vi "Police panel.vi"() -> ()   [LabVIEW 2018]
panel:
  in  "Police Arrived 2":bool
  out "Accident":bool
  in  "Done":bool
  in  "Police Arrived":bool
  in  "Logout":bool
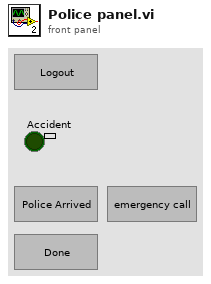
[diagram p1: front panel]
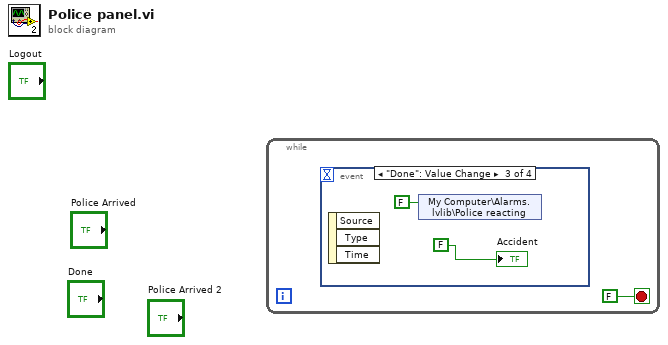
[diagram p0: block diagram]
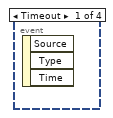
[diagram p2: hidden frame]
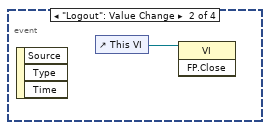
[diagram p3: hidden frame]
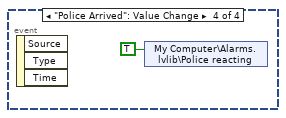
[diagram p4: hidden frame]
diagram:
  n1 = while {
    stop <- FALSE stop-if-true
    n2 = event shown="[2] \"Done\": Value Change" {
      selector: _ -> [_ _ _ _]
      dyn-events: _ -> [_ _ _ _]
      timeout: _ -> [_ _ _ _]
      event Timeout {
        n3 = event-data() -> ()  [unwired: 1 in, 3 out]
      }
      event "Logout": Value Change {
        n4 = event-data() -> ()  [unwired: 1 in, 3 out]
        n5 = control-ref of="This VI"() -> (w2:refnum<vi>)
        n6 = invoke class="VI" method="FP.Close"(reference=w2) -> ()  [unwired: 2 in, 3 out]
      }
      event "Done": Value Change {
        n7 = event-data() -> ()  [unwired: 1 in, 3 out]
        n8 = shared-variable "My Computer\\Alarms.lvlib\\Police reacting"(FALSE ("Repairing")) -> ()  [unwired: 1 in, 1 out]
        "Accident" <- FALSE ("Traffic light failure")
      }
      event "Police Arrived": Value Change {
        n9 = event-data() -> ()  [unwired: 1 in, 3 out]
        n10 = shared-variable "My Computer\\Alarms.lvlib\\Police reacting"(TRUE ("Repairing")) -> ()  [unwired: 1 in, 1 out]
      }
    }
  }
